vi "ExCircBufBin2xTemp.vi"() -> ()   [LabVIEW 2010]
panel:
  out "Thermometer":dbl(slide) min=-150.0 max=0.0 scale format="%.3f"
  in  "Cancel Setting":bool
  out "Temperature Set?":bool
  out "Current Temperature":dbl format="%.2f"
  out "loop cntr":u32
  in  "stop temp loop 1st":bool
  out "Temperature 2":dbl format="%.2f"
  out "Temperature":dbl format="%.2f"
  in  "Software Accumulation":u32=1 min=1 step=1
  in  "Intensifier":bool
  in  "Temperature":dbl=-10.0 format="%.2f"
  in  "Exposure":dbl min=0.0 step=1e-06 format="%.5f"
  in  "Stop Experiment":bool
  in  "Store":bool
  out "error out":errorcluster
  in  "error in (no error)":errorcluster
  # "ExCircBufBin2xTemp: \nThis example only works with cameras with circualar buffer capability. First this routine will set the temperature and wait for it to reach the set point (this can be canceled by pressing the cancel setting stop button. This routine then will continously display an image binned by 2 in both the x and the y direction. It will store in append mode the frames while  the store toggle switch is on. During data acquistion the temperature is \ndisplayed in two different types of loops, one embedded in the data collection and the other in a separate thread.\nThis example should only be run with cameras that have the ability to set the temperature."
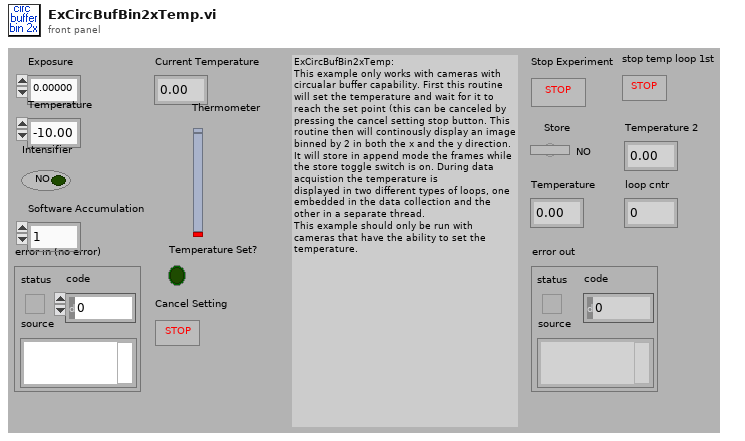
[diagram p1: front panel]
types:
  T1 = cluster{"acquire focus mode":u32, "Exposure":dbl, "Number of Images":u32, "Software Accumulation":u32}
  T2 = cluster{"Camera Handle":u32, "Pulser Handle":u32, "File Handle":u32, "Display Handle":u32, "Image Handle":u32}
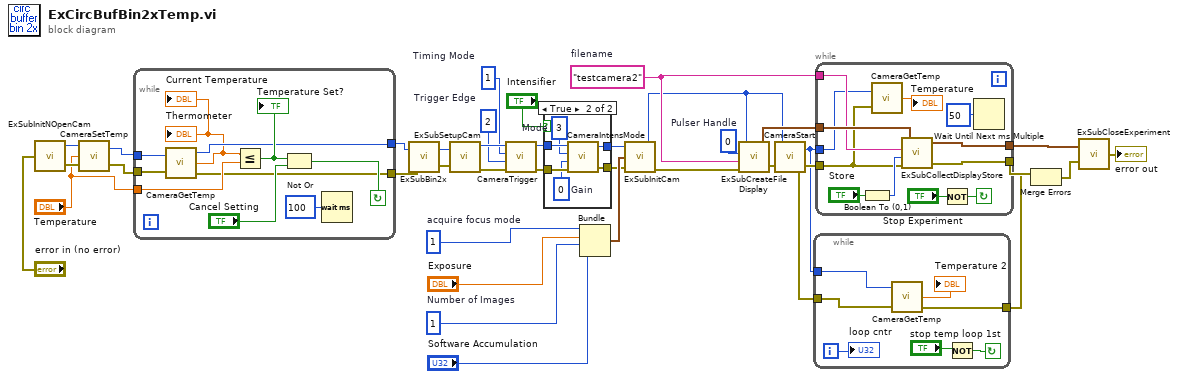
[diagram p0: block diagram]
diagram:
  w20 = u32 0  # Pulser Handle
  w21 = u32 1  # Timing Mode
  w22 = u32 2  # Trigger Edge
  w24 = u32 1  # acquire focus mode
  w23 = u32 1  # Number of Images
  w37 = "testcamera2"  # filename
  n1 = call "ExSubInitNOpenCam.vi"("error in (no error)"="error in (no error)") -> ("Camera Handle"=w12:u32, "error out"=w11:errorcluster)
  n2 = call <userlib>:"CameraSetTemp.vi"("error in (no error)"=w11, "Temperature"="Temperature", "Camera Handle"=w12) -> ("error out"=w7:errorcluster, "Camera Handle"=w8:u32)
  n3 = while {
    tunnel: "Temperature" -> [w47]
    tunnel: w7 -> [w43]
    tunnel: w8 -> [w42]
    tunnel: [w41] -> w5
    tunnel: [w40] -> w4
    stop <- w45 continue-if-true
    n4 = call <userlib>:"CameraGetTemp.vi"("Camera Handle"=w42, "error in (no error)"=w43) -> ("Camera Handle"=w41:u32, "Temperature"=w38:dbl, "error out"=w40:errorcluster)
    "Thermometer" <- w38
    "Current Temperature" <- w38
    n5 = Less Or Equal?(x=w38, y=w47) -> (x <= y?=w44:bool)
    "Temperature Set?" <- w44
    n6 = Not Or(1:"Cancel Setting", 2:w44) -> (0:w45:bool)
    n7 = Wait (ms)(milliseconds to wait=u32 100) -> ()  [unwired: 1 out]
  }
  n8 = call "ExSubBin2x.vi"("error in (no error)"=w4, "Camera Handle"=w5) -> ("error out"=w10:errorcluster, "Camera Handle"=w25:u32)
  n9 = call "ExSubSetupCam.vi"("error in (no error)"=w10, "Camera Handle"=w25) -> ("error out"=w28:errorcluster, "Camera Handle"=w29:u32)
  n10 = call <userlib>:"CameraTrigger.vi"("error in"=w28, "Trigger Edge"=w22, "Timing Mode"=w21, "Camera Handle"=w29) -> ("error out"=w16:errorcluster, "Camera Handle"=w18:u32)
  n11 = case shown="True" "Intensifier" {
    tunnel: w18 -> [w49 w55]
    tunnel: [w49 w54] -> w17
    tunnel: w16 -> [w48 w53]
    tunnel: [w48 w52] -> w15
    frame False {
    }
    frame True {
      w50 = u32 0  # Gain
      w51 = u32 3  # Mode
      n12 = call <userlib>:"CameraIntensMode.vi"("error in"=w53, "Intensifier Gain"=w50, "Mode"=w51, "Camera Handle"=w55) -> ("error out"=w52:errorcluster, "Camera Handle"=w54:u32)
    }
  }
  n13 = Bundle("acquire focus mode"=w24, "Exposure"="Exposure", "Number of Images"=w23, "Software Accumulation"="Software Accumulation") -> (w34:T1)  [unwired: 1 in]
  n14 = call "ExSubInitCam.vi"("error in (no error)"=w15, "Camera Information"=w34, "Camera Handle"=w17) -> ("error out"=w33:errorcluster, "Camera Handle"=w19:u32)
  n15 = call "ExSubCreateFileDisplay.vi"("error in (no error)"=w33, "File and Display Name"=w37, "Pulser Handle"=w20, "Camera Handle"=w19) -> ("error out"=w26:errorcluster, "Handles Out"=w32:T2)
  n16 = call <userlib>:"CameraStart.vi"("error in"=w26, "Camera Handle"=w19) -> ("error out"=w27:errorcluster, "Camera Handle"=w9:u32)
  n17 = while {
    tunnel: w9 -> [w62]
    tunnel: w27 -> [w61]
    tunnel: [w56] -> w2
    i -> [w59]
    stop <- w58 continue-if-true
    n18 = call <userlib>:"CameraGetTemp.vi"("Camera Handle"=w62, "error in (no error)"=w61) -> ("Temperature"=→"Temperature 2":dbl, "error out"=w56:errorcluster)  [unwired: 1 out]
    n19 = Not(x="stop temp loop 1st") -> (.not. x?=w58:bool)
    "loop cntr" <- w59
  }
  n20 = while {
    tunnel: w32 -> [w73]
    tunnel: w27 -> [w65]
    tunnel: w37 -> [w66]
    tunnel: [w71] -> w3
    tunnel: [w72] -> w31
    tunnel: w9 -> [w64]
    stop <- w69 continue-if-true
    n21 = Boolean To (0,1)(Boolean="Store") -> (0, 1=w67:i16)
    n22 = call <userlib>:"CameraGetTemp.vi"("Camera Handle"=w64, "error in (no error)"=w65) -> ("Temperature"=→"Temperature":dbl)  [unwired: 2 out]
    n23 = call "ExSubCollectDisplayStore.vi"("error in (no error)"=w65, "Store flag"=w67, "Display Title"=w66, "Handle Cluster"=w73) -> ("error out"=w71:errorcluster, "Handle Cluster Out"=w72:T2)  [unwired: 1 out]
    n24 = Not(x="Stop Experiment") -> (.not. x?=w69:bool)
    n25 = Wait Until Next ms Multiple(millisecond multiple=u32 50) -> ()  [unwired: 1 out]
  }
  n26 = Merge Errors(w3, w2) -> (w1:errorcluster)
  n27 = call "ExSubCloseExperiment.vi"("error in (no error)"=w1, "Handles In"=w31) -> ("error out"=→"error out":errorcluster)
